vi "Create New Waypoint Dictionary ConfigFile.vi"() -> ()   [LabVIEW 2020, in "WyPtDict.lvlib"]
uses:
  WyPtDict.lvlib
  RoboWaypointDict Node--cluster.ctl
  BRS_Dev/Source Code/Robo Driver/Controls/MC and Robo Handshake.ctl
  StockerExpansionModuleID--enum.ctl
panel:
  out "Error":bool
  out "Nodes Written":i32=78
  out "error out":errorcluster={"status"=TRUE, "code"=10, "source"="Open/Create/Replace File in Easy Write XML File__JKI EasyXML.vi:3150001->Create New Waypoint Dictionary ConfigFile.vi<APPEND>\nC:\\Projects\\BRS-Dev\\BRS Information\\Waypoint Dictionary Configuration File.xml"}
  in  "error in (no error)":errorcluster
  in  "Waypoint Dictionary ConfigFile":path=path "C:/Projects/BRS-Dev/BRS Information/Waypoint Dictionary Configuration File - Template.xml"
  in  "WaypointDictionary":cluster{"WyPtDictNode":T1[]}={"WyPtDictNode"=[{"MC and Robo Handshake"=enum."None", "Idx"=0, "Cmd Number"="", "Waypoint List"="", "Description"="", "ExpMod ID"=enum."None"}, {"MC and Robo Handshake"=enum."Move and Pick Nikon Ret LP(1100)", "Idx"=1, "Cmd Number"="1100", "Waypoint List"="", "Description"="", "ExpMod ID"=enum."None"}, {"MC and Robo Handshake"=enum."Nikon Barcode1 Scanning Started(1101)", "Idx"=2, "Cmd Number"="1101", "Waypoint List"="", "Description"="", "ExpMod ID"=enum."None"}, {"MC and Robo Handshake"=enum."Nikon Barcode1 Scan Abort(1102)", "Idx"=3, "Cmd Number"="1102", "Waypoint List"="", "Description"="", "ExpMod ID"=enum."None"}, {"MC and Robo Handshake"=enum."Nikon Barcode1 Scan Success Proc to Barcode 2 Pos(1103)", "Idx"=4, "Cmd Number"="1103", "Waypoint List"="", "Description"="", "ExpMod ID"=enum."None"}, {"MC and Robo Handshake"=enum."Nikon Barcode 2 Scanning Started(1104)", "Idx"=5, "Cmd Number"="1104", "Waypoint List"="", "Description"="", "ExpMod ID"=enum."None"}, {"MC and Robo Handshake"=enum."Nikon Barcode 2 Scan Abort(1105) ", "Idx"=6, "Cmd Number"="1105", "Waypoint List"="", "Description"="", "ExpMod ID"=enum."None"}, {"MC and Robo Handshake"=enum."Nikon Barcode 2 Success(1106)", "Idx"=7, "Cmd Number"="1106", "Waypoint List"="", "Description"="", "ExpMod ID"=enum."None"}, {"MC and Robo Handshake"=enum."Move and Pick POZZ Ret LP(1300)", "Idx"=8, "Cmd Number"="1300", "Waypoint List"="", "Description"="", "ExpMod ID"=enum."None"}, {"MC and Robo Handshake"=enum."POZZ Barcode Scan Started(1301)", "Idx"=9, "Cmd Number"="1301", "Waypoint List"="", "Description"="", "ExpMod ID"=enum."None"}, {"MC and Robo Handshake"=enum."POZZ Barcode Not Found(1302)", "Idx"=10, "Cmd Number"="1302", "Waypoint List"="", "Description"="", "ExpMod ID"=enum."None"}, {"MC and Robo Handshake"=enum."POZZ Barcode Scan Succ(1303)", "Idx"=11, "Cmd Number"="1303", "Waypoint List"="", "Description"="", "ExpMod ID"=enum."None"}, {"MC and Robo Handshake"=enum."POZZ Mov to Side 2 Bar 2(1310)", "Idx"=12, "Cmd Number"="1310", "Waypoint List"="", "Description"="", "ExpMod ID"=enum."None"}, {"MC and Robo Handshake"=enum."POZZ Mov to Side 4 Bar 1(1311)", "Idx"=13, "Cmd Number"="1311", "Waypoint List"="", "Description"="", "ExpMod ID"=enum."None"}, {"MC and Robo Handshake"=enum."POZZ Mov to Side 4 Bar 2(1312)", "Idx"=14, "Cmd Number"="1312", "Waypoint List"="", "Description"="", "ExpMod ID"=enum."None"}, {"MC and Robo Handshake"=enum."POZZ Mov to Side 1 Bar 1(1313)", "Idx"=15, "Cmd Number"="1313", "Waypoint List"="", "Description"="", "ExpMod ID"=enum."None"}, {"MC and Robo Handshake"=enum."POZZ Mov to Side 1 Bar 2(1314)", "Idx"=16, "Cmd Number"="1314", "Waypoint List"="", "Description"="", "ExpMod ID"=enum."None"}, {"MC and Robo Handshake"=enum."POZZ Mov to Side 3 Bar 1(1315)", "Idx"=17, "Cmd Number"="1315", "Waypoint List"="", "Description"="", "ExpMod ID"=enum."None"}, {"MC and Robo Handshake"=enum."POZZ Mov to Side 3 Bar 2(1316)", "Idx"=18, "Cmd Number"="1316", "Waypoint List"="", "Description"="", "ExpMod ID"=enum."None"}, {"MC and Robo Handshake"=enum."POZZ Mov to Edge 3 Nik 2(1317)", "Idx"=19, "Cmd Number"="1317", "Waypoint List"="", "Description"="", "ExpMod ID"=enum."None"}, {"MC and Robo Handshake"=enum."POZZ Mov to Edge 4 ASML(1318)", "Idx"=20, "Cmd Number"="1318", "Waypoint List"="", "Description"="", "ExpMod ID"=enum."None"}, {"MC and Robo Handshake"=enum."POZZ Mov to Edge 4 Nik 1(1319)", "Idx"=21, "Cmd Number"="1319", "Waypoint List"="", "Description"="", "ExpMod ID"=enum."None"}, {"MC and Robo Handshake"=enum."POZZ Mov to Edge 4 Nik 2(1320)", "Idx"=22, "Cmd Number"="1320", "Waypoint List"="", "Description"="", "ExpMod ID"=enum."None"}, {"MC and Robo Handshake"=enum."Move to ASML LP and Pick Ret(2000)", "Idx"=23, "Cmd Number"="2000", "Waypoint List"="", "Description"="", "ExpMod ID"=enum."None"}, {"MC and Robo Handshake"=enum."ASML1 Barcode Scan Started(2001)", "Idx"=24, "Cmd Number"="2001", "Waypoint List"="", "Description"="", "ExpMod ID"=enum."None"}, {"MC and Robo Handshake"=enum."ASML1 Barcode Not Found(2002)", "Idx"=25, "Cmd Number"="2002", "Waypoint List"="", "Description"="", "ExpMod ID"=enum."None"}, {"MC and Robo Handshake"=enum."ASML1 Barcode Scan Succ(2003)", "Idx"=26, "Cmd Number"="2003", "Waypoint List"="", "Description"="", "ExpMod ID"=enum."None"}, {"MC and Robo Handshake"=enum."Start Load Seq for Nikon LP(3000)", "Idx"=27, "Cmd Number"="3000", "Waypoint List"="", "Description"="", "ExpMod ID"=enum."None"}, {"MC and Robo Handshake"=enum."Start Load Seq for POZZ LP(3200)", "Idx"=28, "Cmd Number"="3200", "Waypoint List"="", "Description"="", "ExpMod ID"=enum."None"}, {"MC and Robo Handshake"=enum."Start Load Seq for ASML LP(3400)", "Idx"=29, "Cmd Number"="3400", "Waypoint List"="", "Description"="", "ExpMod ID"=enum."None"}, {"MC and Robo Handshake"=enum."Start Align End Grip Place Func(4000)", "Idx"=30, "Cmd Number"="4000", "Waypoint List"="", "Description"="", "ExpMod ID"=enum."None"}, {"MC and Robo Handshake"=enum."Start Align End grip Pick Func(4001)", "Idx"=31, "Cmd Number"="4001", "Waypoint List"="", "Description"="", "ExpMod ID"=enum."None"}, {"MC and Robo Handshake"=enum."Start Align Center Grip Place Func(4002)", "Idx"=32, "Cmd Number"="4002", "Waypoint List"="", "Description"="", "ExpMod ID"=enum."None"}, {"MC and Robo Handshake"=enum."Start Align Center grip Pick Func(4003)", "Idx"=33, "Cmd Number"="4003", "Waypoint List"="", "Description"="", "ExpMod ID"=enum."None"}, {"MC and Robo Handshake"=enum."Start Move from home to Cleaner(5000)", "Idx"=34, "Cmd Number"="5000", "Waypoint List"="", "Description"="", "ExpMod ID"=enum."None"}, {"MC and Robo Handshake"=enum."Start Move to Final Cleaner Loc(5001)", "Idx"=35, "Cmd Number"="5001", "Waypoint List"="", "Description"="", "ExpMod ID"=enum."None"}, {"MC and Robo Handshake"=enum."Start Move from Cleaner loc to home(5002)", "Idx"=36, "Cmd Number"="5002", "Waypoint List"="", "Description"="", "ExpMod ID"=enum."None"}, {"MC and Robo Handshake"=enum."Start Move from home to PDS for Inspect(6000) ", "Idx"=37, "Cmd Number"="6000", "Waypoint List"="", "Description"="", "ExpMod ID"=enum."None"}, {"MC and Robo Handshake"=enum."PDS Inspect Finished(6001)", "Idx"=38, "Cmd Number"="6001", "Waypoint List"="", "Description"="", "ExpMod ID"=enum."None"}, {"MC and Robo Handshake"=enum."PDS EMO Recovery(6002)", "Idx"=39, "Cmd Number"="6002", "Waypoint List"="", "Description"="", "ExpMod ID"=enum."None"}, {"MC and Robo Handshake"=enum."Store in Stocker(7001)", "Idx"=40, "Cmd Number"="7001", "Waypoint List"="", "Description"="", "ExpMod ID"=enum."None"}, {"MC and Robo Handshake"=enum."Store in Expansion Stocker(7402)", "Idx"=41, "Cmd Number"="7401", "Waypoint List"="", "Description"="", "ExpMod ID"=enum."None"}, {"MC and Robo Handshake"=enum."Retrive from Center Stocker(8001)", "Idx"=42, "Cmd Number"="8001", "Waypoint List"="", "Description"="", "ExpMod ID"=enum."None"}, {"MC and Robo Handshake"=enum."Retrive Mov to Nikon BC1 Scan Pos(8002)", "Idx"=43, "Cmd Number"="8002", "Waypoint List"="", "Description"="", "ExpMod ID"=enum."None"}, {"MC and Robo Handshake"=enum."Retrive Nikon BC1not found(8003)", "Idx"=44, "Cmd Number"="8003", "Waypoint List"="", "Description"="", "ExpMod ID"=enum."None"}, {"MC and Robo Handshake"=enum."Retrive Nikon BC1 Scan Succ(8004)", "Idx"=45, "Cmd Number"="8004", "Waypoint List"="", "Description"="", "ExpMod ID"=enum."None"}, {"MC and Robo Handshake"=enum."Retrive Nikon BC2 not found(8005)", "Idx"=46, "Cmd Number"="8005", "Waypoint List"="", "Description"="", "ExpMod ID"=enum."None"}, {"MC and Robo Handshake"=enum."Retrive Nikon BC2 scan Succ(8006)", "Idx"=47, "Cmd Number"="8006", "Waypoint List"="", "Description"="", "ExpMod ID"=enum."None"}, {"MC and Robo Handshake"=enum."Retrive Mov to Edge 1 ASML(8202) ", "Idx"=48, "Cmd Number"="8202", "Waypoint List"="", "Description"="", "ExpMod ID"=enum."None"}, {"MC and Robo Handshake"=enum."Retrive Mov to Edge 1 Nikon 1(8203)", "Idx"=49, "Cmd Number"="8203", "Waypoint List"="", "Description"="", "ExpMod ID"=enum."None"}, {"MC and Robo Handshake"=enum."Retrive Mov to Edge 1 Nikon 2(8204)", "Idx"=50, "Cmd Number"="8204", "Waypoint List"="", "Description"="", "ExpMod ID"=enum."None"}, {"MC and Robo Handshake"=enum."Retrive Mov to Edge 2 ASML(8205)", "Idx"=51, "Cmd Number"="8205", "Waypoint List"="", "Description"="", "ExpMod ID"=enum."None"}, {"MC and Robo Handshake"=enum."Retrive Mov to Edge 2 Nikon 1(8206)", "Idx"=52, "Cmd Number"="8206", "Waypoint List"="", "Description"="", "ExpMod ID"=enum."None"}, {"MC and Robo Handshake"=enum."Retrive Mov to Edge 2 Nikon 2(8207)", "Idx"=53, "Cmd Number"="8207", "Waypoint List"="", "Description"="", "ExpMod ID"=enum."None"}, {"MC and Robo Handshake"=enum."Retrive Mov to Edge 3 ASML (8208)", "Idx"=54, "Cmd Number"="8208", "Waypoint List"="", "Description"="", "ExpMod ID"=enum."None"}, {"MC and Robo Handshake"=enum."Retrive Mov to Edge 3 Nikon 1(8209)", "Idx"=55, "Cmd Number"="8209", "Waypoint List"="", "Description"="", "ExpMod ID"=enum."None"}, {"MC and Robo Handshake"=enum."Retrive Mov to Edge 3 Nikon 2(8210)", "Idx"=56, "Cmd Number"="8210", "Waypoint List"="", "Description"="", "ExpMod ID"=enum."None"}, {"MC and Robo Handshake"=enum."Retrive Mov to Edge 4 ASML (8211)", "Idx"=57, "Cmd Number"="8211", "Waypoint List"="", "Description"="", "ExpMod ID"=enum."None"}, {"MC and Robo Handshake"=enum."Retrive Mov to Edge 4 Nikon 1 (8212)", "Idx"=58, "Cmd Number"="8212", "Waypoint List"="", "Description"="", "ExpMod ID"=enum."None"}, {"MC and Robo Handshake"=enum."Retrive Mov to Edge 4 Nikon 2 (8213)", "Idx"=59, "Cmd Number"="8213", "Waypoint List"="", "Description"="", "ExpMod ID"=enum."None"}, {"MC and Robo Handshake"=enum."Retrive BC Scan Abort (8214)", "Idx"=60, "Cmd Number"="8214", "Waypoint List"="", "Description"="", "ExpMod ID"=enum."None"}, {"MC and Robo Handshake"=enum."Retrive BC Scan Successful (8215)", "Idx"=61, "Cmd Number"="8215", "Waypoint List"="", "Description"="", "ExpMod ID"=enum."None"}, {"MC and Robo Handshake"=enum."Retrive Mov to ASML BC scan Pos (8402) ", "Idx"=62, "Cmd Number"="8402", "Waypoint List"="", "Description"="", "ExpMod ID"=enum."None"}, {"MC and Robo Handshake"=enum."Retrive ASML BC not found(8403)", "Idx"=63, "Cmd Number"="8403", "Waypoint List"="", "Description"="", "ExpMod ID"=enum."None"}, {"MC and Robo Handshake"=enum."Retrive ASML BC Scan Succ(8404)", "Idx"=64, "Cmd Number"="8404", "Waypoint List"="", "Description"="", "ExpMod ID"=enum."None"}, {"MC and Robo Handshake"=enum."Expansion Retrive Seq (8602)", "Idx"=65, "Cmd Number"="8601", "Waypoint List"="", "Description"="", "ExpMod ID"=enum."None"}, {"MC and Robo Handshake"=enum."Cen Stocker move from home to Transit Nest(9000)", "Idx"=66, "Cmd Number"="9000", "Waypoint List"="", "Description"="", "ExpMod ID"=enum."None"}, {"MC and Robo Handshake"=enum."Cen Stocker move from Transit Nest to home(9200)", "Idx"=67, "Cmd Number"="9200", "Waypoint List"="", "Description"="", "ExpMod ID"=enum."None"}, {"MC and Robo Handshake"=enum."Exp Stocker move from home to Transit Nest(9400)", "Idx"=68, "Cmd Number"="9400", "Waypoint List"="", "Description"="", "ExpMod ID"=enum."None"}, {"MC and Robo Handshake"=enum."Exp Stocker move from Transit Nest to home(9600)", "Idx"=69, "Cmd Number"="9600", "Waypoint List"="", "Description"="", "ExpMod ID"=enum."None"}, {"MC and Robo Handshake"=enum."Move to R1 Home (1000)", "Idx"=70, "Cmd Number"="1000", "Waypoint List"="", "Description"="", "ExpMod ID"=enum."None"}, {"MC and Robo Handshake"=enum."Move to R2 Home (1111)", "Idx"=71, "Cmd Number"="1000", "Waypoint List"="", "Description"="", "ExpMod ID"=enum."None"}, {"MC and Robo Handshake"=enum."Store Left Stocker (7401)", "Idx"=72, "Cmd Number"="7401", "Waypoint List"="", "Description"="", "ExpMod ID"=enum."None"}, {"MC and Robo Handshake"=enum."Retrieve Left Stocker (8601)", "Idx"=73, "Cmd Number"="8601", "Waypoint List"="", "Description"="", "ExpMod ID"=enum."None"}, {"MC and Robo Handshake"=enum."EMO Recovery Center (1002)", "Idx"=74, "Cmd Number"="1002", "Waypoint List"="", "Description"="", "ExpMod ID"=enum."None"}, {"MC and Robo Handshake"=enum."EMO Recovery Right (1003)", "Idx"=75, "Cmd Number"="1002", "Waypoint List"="", "Description"="", "ExpMod ID"=enum."None"}, {"MC and Robo Handshake"=enum."Center Robo Status (8888)", "Idx"=76, "Cmd Number"="8888", "Waypoint List"="", "Description"="", "ExpMod ID"=enum."None"}, {"MC and Robo Handshake"=enum."Right Robo Status (8889)", "Idx"=77, "Cmd Number"="8888", "Waypoint List"="", "Description"="", "ExpMod ID"=enum."None"}]}
  # "XML Configuration File"
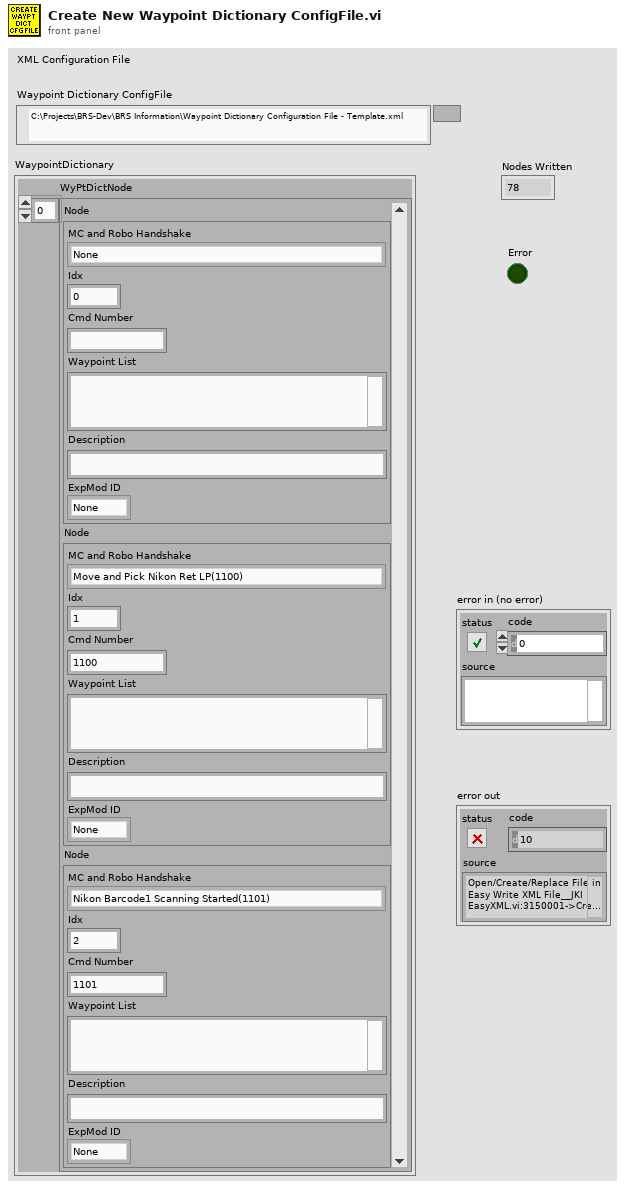
[diagram p1: front panel]
types:
  T1 = typedef "WyPtDict.lvlib/RoboWaypointDict Node--cluster.ctl" = cluster{"MC and Robo Handshake":T2, "Idx":i32, "Cmd Number":string, "Waypoint List":string, "Description":string, "ExpMod ID":T3}
  T2 = typedef "MC and Robo Handshake.ctl" = enum16{"None", "Move and Pick Nikon Ret LP(1100)", "Nikon Barcode1 Scanning Started(1101)", "Nikon Barcode1 Scan Abort(1102)", "Nikon Barcode1 Scan Success Proc to Barcode 2 Pos(1103)", "Nikon Barcode 2 Scanning Started(1104)", "Nikon Barcode 2 Scan Abort(1105) ", "Nikon Barcode 2 Success(1106)", "Move and Pick POZZ Ret LP(1300)", "POZZ Barcode Scan Started(1301)", "POZZ Barcode Not Found(1302)", "POZZ Barcode Scan Succ(1303)", "POZZ Mov to Side 2 Bar 2(1310)", "POZZ Mov to Side 4 Bar 1(1311)", "POZZ Mov to Side 4 Bar 2(1312)", "POZZ Mov to Side 1 Bar 1(1313)", "POZZ Mov to Side 1 Bar 2(1314)", "POZZ Mov to Side 3 Bar 1(1315)", "POZZ Mov to Side 3 Bar 2(1316)", "POZZ Mov to Edge 3 Nik 2(1317)", "POZZ Mov to Edge 4 ASML(1318)", "POZZ Mov to Edge 4 Nik 1(1319)", "POZZ Mov to Edge 4 Nik 2(1320)", "Move to ASML LP and Pick Ret(2000)", "ASML1 Barcode Scan Started(2001)", "ASML1 Barcode Not Found(2002)", "ASML1 Barcode Scan Succ(2003)", "Start Load Seq for Nikon LP(3000)", "Start Load Seq for POZZ LP(3200)", "Start Load Seq for ASML LP(3400)", "Start Align End Grip Place Func(4000)", "Start Align End grip Pick Func(4001)", "Start Align Center Grip Place Func(4002)", "Start Align Center grip Pick Func(4003)", "Start Move from home to Cleaner(5000)", "Start Move to Final Cleaner Loc(5001)", "Start Move from Cleaner loc to home(5002)", "Start Move from home to PDS for Inspect(6000) ", "PDS Inspect Finished(6001)", "PDS EMO Recovery(6002)", "Store in Stocker(7001)", "Store in Expansion Stocker(7402)", "Retrive from Center Stocker(8001)", "Retrive Mov to Nikon BC1 Scan Pos(8002)", "Retrive Nikon BC1not found(8003)", "Retrive Nikon BC1 Scan Succ(8004)", "Retrive Nikon BC2 not found(8005)", "Retrive Nikon BC2 scan Succ(8006)", "Retrive Mov to Edge 1 ASML(8202) ", "Retrive Mov to Edge 1 Nikon 1(8203)", "Retrive Mov to Edge 1 Nikon 2(8204)", "Retrive Mov to Edge 2 ASML(8205)", "Retrive Mov to Edge 2 Nikon 1(8206)", "Retrive Mov to Edge 2 Nikon 2(8207)", "Retrive Mov to Edge 3 ASML (8208)", "Retrive Mov to Edge 3 Nikon 1(8209)", "Retrive Mov to Edge 3 Nikon 2(8210)", "Retrive Mov to Edge 4 ASML (8211)", "Retrive Mov to Edge 4 Nikon 1 (8212)", "Retrive Mov to Edge 4 Nikon 2 (8213)", "Retrive BC Scan Abort (8214)", "Retrive BC Scan Successful (8215)", "Retrive Mov to ASML BC scan Pos (8402) ", "Retrive ASML BC not found(8403)", "Retrive ASML BC Scan Succ(8404)", "Expansion Retrive Seq (8602)", "Cen Stocker move from home to Transit Nest(9000)", "Cen Stocker move from Transit Nest to home(9200)", "Exp Stocker move from home to Transit Nest(9400)", "Exp Stocker move from Transit Nest to home(9600)", "Move to R1 Home (1000)", "Move to R2 Home (1111)", "Store Left Stocker (7401)", "Retrieve Left Stocker (8601)", "EMO Recovery Center (1002)", "EMO Recovery Right (1003)", "Center Robo Status (8888)", "Right Robo Status (8889)"}
  T3 = typedef "WyPtDict.lvlib/StockerExpansionModuleID--enum.ctl" = enum16{"None", "Main", "Exp1", "Exp2", "Exp3", "Exp4", "Exp5"}
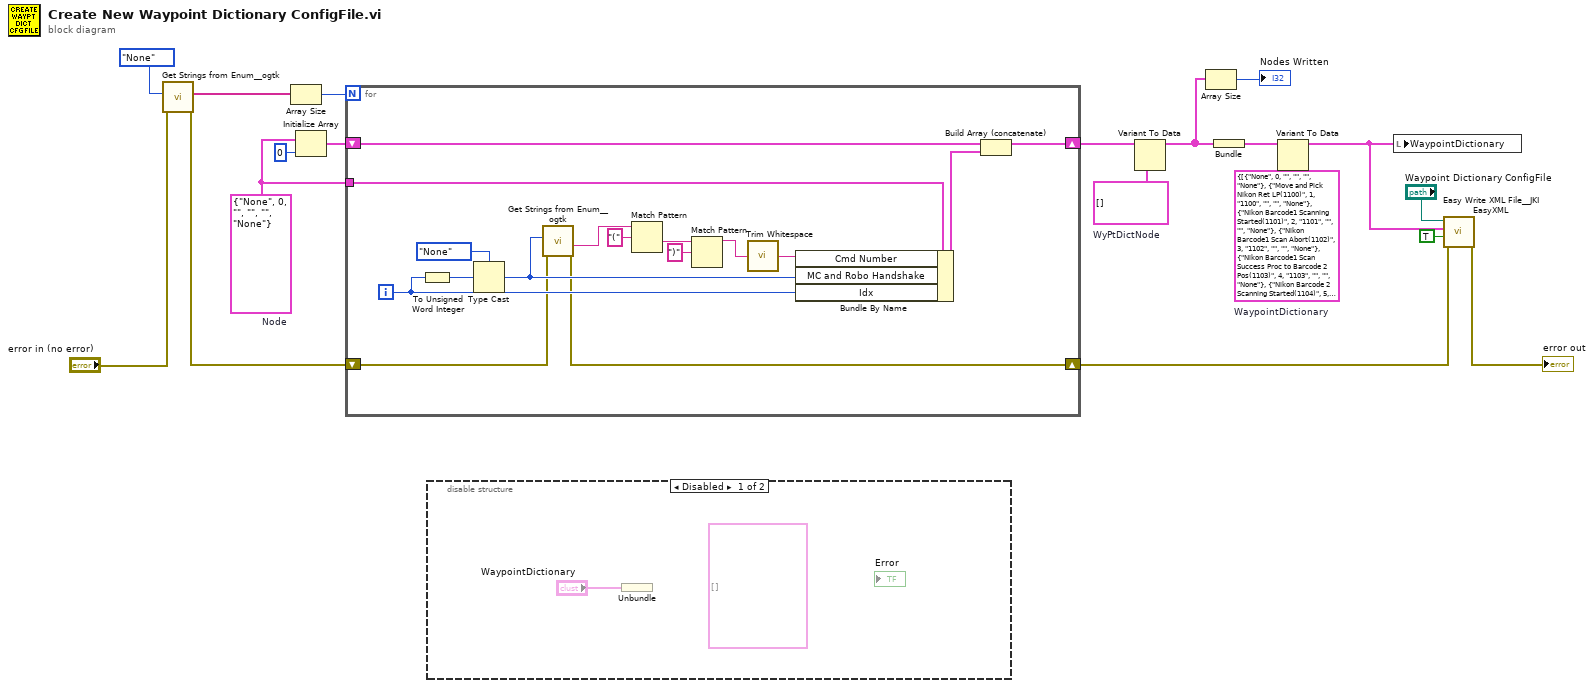
[diagram p0: block diagram]
diagram:
  w2 = cluster{"WyPtDictNode":T1[]} {"WyPtDictNode"=[{"MC and Robo Handshake"=enum."None", "Idx"=0, "Cmd Number"="", "Waypoint List"="", "Description"="", "ExpMod ID"=enum."None"}, {"MC and Robo Handshake"=enum."Move and Pick Nikon Ret LP(1100)", "Idx"=1, "Cmd Number"="1100", "Waypoint List"="", "Description"="", "ExpMod ID"=enum."None"}, {"MC and Robo Handshake"=enum."Nikon Barcode1 Scanning Started(1101)", "Idx"=2, "Cmd Number"="1101", "Waypoint List"="", "Description"="", "ExpMod ID"=enum."None"}, {"MC and Robo Handshake"=enum."Nikon Barcode1 Scan Abort(1102)", "Idx"=3, "Cmd Number"="1102", "Waypoint List"="", "Description"="", "ExpMod ID"=enum."None"}, {"MC and Robo Handshake"=enum."Nikon Barcode1 Scan Success Proc to Barcode 2 Pos(1103)", "Idx"=4, "Cmd Number"="1103", "Waypoint List"="", "Description"="", "ExpMod ID"=enum."None"}, {"MC and Robo Handshake"=enum."Nikon Barcode 2 Scanning Started(1104)", "Idx"=5, "Cmd Number"="1104", "Waypoint List"="", "Description"="", "ExpMod ID"=enum."None"}, {"MC and Robo Handshake"=enum."Nikon Barcode 2 Scan Abort(1105) ", "Idx"=6, "Cmd Number"="1105", "Waypoint List"="", "Description"="", "ExpMod ID"=enum."None"}, {"MC and Robo Handshake"=enum."Nikon Barcode 2 Success(1106)", "Idx"=7, "Cmd Number"="1106", "Waypoint List"="", "Description"="", "ExpMod ID"=enum."None"}, {"MC and Robo Handshake"=enum."Move and Pick POZZ Ret LP(1300)", "Idx"=8, "Cmd Number"="1300", "Waypoint List"="", "Description"="", "ExpMod ID"=enum."None"}, {"MC and Robo Handshake"=enum."POZZ Barcode Scan Started(1301)", "Idx"=9, "Cmd Number"="1301", "Waypoint List"="", "Description"="", "ExpMod ID"=enum."None"}, {"MC and Robo Handshake"=enum."POZZ Barcode Not Found(1302)", "Idx"=10, "Cmd Number"="1302", "Waypoint List"="", "Description"="", "ExpMod ID"=enum."None"}, {"MC and Robo Handshake"=enum."POZZ Barcode Scan Succ(1303)", "Idx"=11, "Cmd Number"="1303", "Waypoint List"="", "Description"="", "ExpMod ID"=enum."None"}, {"MC and Robo Handshake"=enum."POZZ Mov to Side 2 Bar 2(1310)", "Idx"=12, "Cmd Number"="1310", "Waypoint List"="", "Description"="", "ExpMod ID"=enum."None"}, {"MC and Robo Handshake"=enum."POZZ Mov to Side 4 Bar 1(1311)", "Idx"=13, "Cmd Number"="1311", "Waypoint List"="", "Description"="", "ExpMod ID"=enum."None"}, {"MC and Robo Handshake"=enum."POZZ Mov to Side 4 Bar 2(1312)", "Idx"=14, "Cmd Number"="1312", "Waypoint List"="", "Description"="", "ExpMod ID"=enum."None"}, {"MC and Robo Handshake"=enum."POZZ Mov to Side 1 Bar 1(1313)", "Idx"=15, "Cmd Number"="1313", "Waypoint List"="", "Description"="", "ExpMod ID"=enum."None"}, {"MC and Robo Handshake"=enum."POZZ Mov to Side 1 Bar 2(1314)", "Idx"=16, "Cmd Number"="1314", "Waypoint List"="", "Description"="", "ExpMod ID"=enum."None"}, {"MC and Robo Handshake"=enum."POZZ Mov to Side 3 Bar 1(1315)", "Idx"=17, "Cmd Number"="1315", "Waypoint List"="", "Description"="", "ExpMod ID"=enum."None"}, {"MC and Robo Handshake"=enum."POZZ Mov to Side 3 Bar 2(1316)", "Idx"=18, "Cmd Number"="1316", "Waypoint List"="", "Description"="", "ExpMod ID"=enum."None"}, {"MC and Robo Handshake"=enum."POZZ Mov to Edge 3 Nik 2(1317)", "Idx"=19, "Cmd Number"="1317", "Waypoint List"="", "Description"="", "ExpMod ID"=enum."None"}, {"MC and Robo Handshake"=enum."POZZ Mov to Edge 4 ASML(1318)", "Idx"=20, "Cmd Number"="1318", "Waypoint List"="", "Description"="", "ExpMod ID"=enum."None"}, {"MC and Robo Handshake"=enum."POZZ Mov to Edge 4 Nik 1(1319)", "Idx"=21, "Cmd Number"="1319", "Waypoint List"="", "Description"="", "ExpMod ID"=enum."None"}, {"MC and Robo Handshake"=enum."POZZ Mov to Edge 4 Nik 2(1320)", "Idx"=22, "Cmd Number"="1320", "Waypoint List"="", "Description"="", "ExpMod ID"=enum."None"}, {"MC and Robo Handshake"=enum."Move to ASML LP and Pick Ret(2000)", "Idx"=23, "Cmd Number"="2000", "Waypoint List"="", "Description"="", "ExpMod ID"=enum."None"}, {"MC and Robo Handshake"=enum."ASML1 Barcode Scan Started(2001)", "Idx"=24, "Cmd Number"="2001", "Waypoint List"="", "Description"="", "ExpMod ID"=enum."None"}, {"MC and Robo Handshake"=enum."ASML1 Barcode Not Found(2002)", "Idx"=25, "Cmd Number"="2002", "Waypoint List"="", "Description"="", "ExpMod ID"=enum."None"}, {"MC and Robo Handshake"=enum."ASML1 Barcode Scan Succ(2003)", "Idx"=26, "Cmd Number"="2003", "Waypoint List"="", "Description"="", "ExpMod ID"=enum."None"}, {"MC and Robo Handshake"=enum."Start Load Seq for Nikon LP(3000)", "Idx"=27, "Cmd Number"="3000", "Waypoint List"="", "Description"="", "ExpMod ID"=enum."None"}, {"MC and Robo Handshake"=enum."Start Load Seq for POZZ LP(3200)", "Idx"=28, "Cmd Number"="3200", "Waypoint List"="", "Description"="", "ExpMod ID"=enum."None"}, {"MC and Robo Handshake"=enum."Start Load Seq for ASML LP(3400)", "Idx"=29, "Cmd Number"="3400", "Waypoint List"="", "Description"="", "ExpMod ID"=enum."None"}, {"MC and Robo Handshake"=enum."Start Align End Grip Place Func(4000)", "Idx"=30, "Cmd Number"="4000", "Waypoint List"="", "Description"="", "ExpMod ID"=enum."None"}, {"MC and Robo Handshake"=enum."Start Align End grip Pick Func(4001)", "Idx"=31, "Cmd Number"="4001", "Waypoint List"="", "Description"="", "ExpMod ID"=enum."None"}, {"MC and Robo Handshake"=enum."Start Align Center Grip Place Func(4002)", "Idx"=32, "Cmd Number"="4002", "Waypoint List"="", "Description"="", "ExpMod ID"=enum."None"}, {"MC and Robo Handshake"=enum."Start Align Center grip Pick Func(4003)", "Idx"=33, "Cmd Number"="4003", "Waypoint List"="", "Description"="", "ExpMod ID"=enum."None"}, {"MC and Robo Handshake"=enum."Start Move from home to Cleaner(5000)", "Idx"=34, "Cmd Number"="5000", "Waypoint List"="", "Description"="", "ExpMod ID"=enum."None"}, {"MC and Robo Handshake"=enum."Start Move to Final Cleaner Loc(5001)", "Idx"=35, "Cmd Number"="5001", "Waypoint List"="", "Description"="", "ExpMod ID"=enum."None"}, {"MC and Robo Handshake"=enum."Start Move from Cleaner loc to home(5002)", "Idx"=36, "Cmd Number"="5002", "Waypoint List"="", "Description"="", "ExpMod ID"=enum."None"}, {"MC and Robo Handshake"=enum."Start Move from home to PDS for Inspect(6000) ", "Idx"=37, "Cmd Number"="6000", "Waypoint List"="", "Description"="", "ExpMod ID"=enum."None"}, {"MC and Robo Handshake"=enum."PDS Inspect Finished(6001)", "Idx"=38, "Cmd Number"="6001", "Waypoint List"="", "Description"="", "ExpMod ID"=enum."None"}, {"MC and Robo Handshake"=enum."PDS EMO Recovery(6002)", "Idx"=39, "Cmd Number"="6002", "Waypoint List"="", "Description"="", "ExpMod ID"=enum."None"}, {"MC and Robo Handshake"=enum."Store in Stocker(7001)", "Idx"=40, "Cmd Number"="7001", "Waypoint List"="", "Description"="", "ExpMod ID"=enum."None"}, {"MC and Robo Handshake"=enum."Store in Expansion Stocker(7402)", "Idx"=41, "Cmd Number"="7401", "Waypoint List"="", "Description"="", "ExpMod ID"=enum."None"}, {"MC and Robo Handshake"=enum."Retrive from Center Stocker(8001)", "Idx"=42, "Cmd Number"="8001", "Waypoint List"="", "Description"="", "ExpMod ID"=enum."None"}, {"MC and Robo Handshake"=enum."Retrive Mov to Nikon BC1 Scan Pos(8002)", "Idx"=43, "Cmd Number"="8002", "Waypoint List"="", "Description"="", "ExpMod ID"=enum."None"}, {"MC and Robo Handshake"=enum."Retrive Nikon BC1not found(8003)", "Idx"=44, "Cmd Number"="8003", "Waypoint List"="", "Description"="", "ExpMod ID"=enum."None"}, {"MC and Robo Handshake"=enum."Retrive Nikon BC1 Scan Succ(8004)", "Idx"=45, "Cmd Number"="8004", "Waypoint List"="", "Description"="", "ExpMod ID"=enum."None"}, {"MC and Robo Handshake"=enum."Retrive Nikon BC2 not found(8005)", "Idx"=46, "Cmd Number"="8005", "Waypoint List"="", "Description"="", "ExpMod ID"=enum."None"}, {"MC and Robo Handshake"=enum."Retrive Nikon BC2 scan Succ(8006)", "Idx"=47, "Cmd Number"="8006", "Waypoint List"="", "Description"="", "ExpMod ID"=enum."None"}, {"MC and Robo Handshake"=enum."Retrive Mov to Edge 1 ASML(8202) ", "Idx"=48, "Cmd Number"="8202", "Waypoint List"="", "Description"="", "ExpMod ID"=enum."None"}, {"MC and Robo Handshake"=enum."Retrive Mov to Edge 1 Nikon 1(8203)", "Idx"=49, "Cmd Number"="8203", "Waypoint List"="", "Description"="", "ExpMod ID"=enum."None"}, {"MC and Robo Handshake"=enum."Retrive Mov to Edge 1 Nikon 2(8204)", "Idx"=50, "Cmd Number"="8204", "Waypoint List"="", "Description"="", "ExpMod ID"=enum."None"}, {"MC and Robo Handshake"=enum."Retrive Mov to Edge 2 ASML(8205)", "Idx"=51, "Cmd Number"="8205", "Waypoint List"="", "Description"="", "ExpMod ID"=enum."None"}, {"MC and Robo Handshake"=enum."Retrive Mov to Edge 2 Nikon 1(8206)", "Idx"=52, "Cmd Number"="8206", "Waypoint List"="", "Description"="", "ExpMod ID"=enum."None"}, {"MC and Robo Handshake"=enum."Retrive Mov to Edge 2 Nikon 2(8207)", "Idx"=53, "Cmd Number"="8207", "Waypoint List"="", "Description"="", "ExpMod ID"=enum."None"}, {"MC and Robo Handshake"=enum."Retrive Mov to Edge 3 ASML (8208)", "Idx"=54, "Cmd Number"="8208", "Waypoint List"="", "Description"="", "ExpMod ID"=enum."None"}, {"MC and Robo Handshake"=enum."Retrive Mov to Edge 3 Nikon 1(8209)", "Idx"=55, "Cmd Number"="8209", "Waypoint List"="", "Description"="", "ExpMod ID"=enum."None"}, {"MC and Robo Handshake"=enum."Retrive Mov to Edge 3 Nikon 2(8210)", "Idx"=56, "Cmd Number"="8210", "Waypoint List"="", "Description"="", "ExpMod ID"=enum."None"}, {"MC and Robo Handshake"=enum."Retrive Mov to Edge 4 ASML (8211)", "Idx"=57, "Cmd Number"="8211", "Waypoint List"="", "Description"="", "ExpMod ID"=enum."None"}, {"MC and Robo Handshake"=enum."Retrive Mov to Edge 4 Nikon 1 (8212)", "Idx"=58, "Cmd Number"="8212", "Waypoint List"="", "Description"="", "ExpMod ID"=enum."None"}, {"MC and Robo Handshake"=enum."Retrive Mov to Edge 4 Nikon 2 (8213)", "Idx"=59, "Cmd Number"="8213", "Waypoint List"="", "Description"="", "ExpMod ID"=enum."None"}, {"MC and Robo Handshake"=enum."Retrive BC Scan Abort (8214)", "Idx"=60, "Cmd Number"="8214", "Waypoint List"="", "Description"="", "ExpMod ID"=enum."None"}, {"MC and Robo Handshake"=enum."Retrive BC Scan Successful (8215)", "Idx"=61, "Cmd Number"="8215", "Waypoint List"="", "Description"="", "ExpMod ID"=enum."None"}, {"MC and Robo Handshake"=enum."Retrive Mov to ASML BC scan Pos (8402) ", "Idx"=62, "Cmd Number"="8402", "Waypoint List"="", "Description"="", "ExpMod ID"=enum."None"}, {"MC and Robo Handshake"=enum."Retrive ASML BC not found(8403)", "Idx"=63, "Cmd Number"="8403", "Waypoint List"="", "Description"="", "ExpMod ID"=enum."None"}, {"MC and Robo Handshake"=enum."Retrive ASML BC Scan Succ(8404)", "Idx"=64, "Cmd Number"="8404", "Waypoint List"="", "Description"="", "ExpMod ID"=enum."None"}, {"MC and Robo Handshake"=enum."Expansion Retrive Seq (8602)", "Idx"=65, "Cmd Number"="8601", "Waypoint List"="", "Description"="", "ExpMod ID"=enum."None"}, {"MC and Robo Handshake"=enum."Cen Stocker move from home to Transit Nest(9000)", "Idx"=66, "Cmd Number"="9000", "Waypoint List"="", "Description"="", "ExpMod ID"=enum."None"}, {"MC and Robo Handshake"=enum."Cen Stocker move from Transit Nest to home(9200)", "Idx"=67, "Cmd Number"="9200", "Waypoint List"="", "Description"="", "ExpMod ID"=enum."None"}, {"MC and Robo Handshake"=enum."Exp Stocker move from home to Transit Nest(9400)", "Idx"=68, "Cmd Number"="9400", "Waypoint List"="", "Description"="", "ExpMod ID"=enum."None"}, {"MC and Robo Handshake"=enum."Exp Stocker move from Transit Nest to home(9600)", "Idx"=69, "Cmd Number"="9600", "Waypoint List"="", "Description"="", "ExpMod ID"=enum."None"}, {"MC and Robo Handshake"=enum."Move to R1 Home (1000)", "Idx"=70, "Cmd Number"="1000", "Waypoint List"="", "Description"="", "ExpMod ID"=enum."None"}, {"MC and Robo Handshake"=enum."Move to R2 Home (1111)", "Idx"=71, "Cmd Number"="1000", "Waypoint List"="", "Description"="", "ExpMod ID"=enum."None"}, {"MC and Robo Handshake"=enum."Store Left Stocker (7401)", "Idx"=72, "Cmd Number"="7401", "Waypoint List"="", "Description"="", "ExpMod ID"=enum."None"}, {"MC and Robo Handshake"=enum."Retrieve Left Stocker (8601)", "Idx"=73, "Cmd Number"="8601", "Waypoint List"="", "Description"="", "ExpMod ID"=enum."None"}, {"MC and Robo Handshake"=enum."EMO Recovery Center (1002)", "Idx"=74, "Cmd Number"="1002", "Waypoint List"="", "Description"="", "ExpMod ID"=enum."None"}, {"MC and Robo Handshake"=enum."EMO Recovery Right (1003)", "Idx"=75, "Cmd Number"="1002", "Waypoint List"="", "Description"="", "ExpMod ID"=enum."None"}, {"MC and Robo Handshake"=enum."Center Robo Status (8888)", "Idx"=76, "Cmd Number"="8888", "Waypoint List"="", "Description"="", "ExpMod ID"=enum."None"}, {"MC and Robo Handshake"=enum."Right Robo Status (8889)", "Idx"=77, "Cmd Number"="8888", "Waypoint List"="", "Description"="", "ExpMod ID"=enum."None"}]}  # WaypointDictionary
  w3 = T1[] []  # WyPtDictNode
  w15 = T1 {"MC and Robo Handshake"=enum."None", "Idx"=0, "Cmd Number"="", "Waypoint List"="", "Description"="", "ExpMod ID"=enum."None"}  # Node
  n1 = call <userlib>:"Get Strings from Enum__ogtk.vi"("error in (no error)"="error in (no error)", "Enum"=MC_and_Robo_Handshake."None" ("MC and Robo Handshake")) -> ("error out"=w11:errorcluster, "Enum Strings"=w17:string[])  [unwired: 6 in, 2 out]
  n2 = Array Size(array=w17) -> (size(s)=w14:i32)
  n3 = Initialize Array(w15, 0 ("dimension size")) -> (w19:T1[])
  n4 = for {
    N: w14 -> [_]
    shift-right: [w31] -> w4
    shift-left: w19 -> [w33]
    tunnel: w15 -> [w34]
    shift-right: [w22] -> w8
    shift-left: w11 -> [w23]
    i -> [w30]
    n5 = To Unsigned Word Integer(number=w30) -> (unsigned 16bit integer=w29:u16)
    n6 = Type Cast(type=MC_and_Robo_Handshake."None" ("MC and Robo Handshake"), x=w29) -> (*(type *) &x=w28:T2)
    n7 = call <userlib>:"Get Strings from Enum__ogtk.vi"("error in (no error)"=w23, "Enum"=w28) -> ("error out"=w22:errorcluster, "String Value"=w21:string)  [unwired: 6 in, 2 out]
    n8 = Match Pattern(string=w21, regular expression="(") -> (after substring=w26:string)  [unwired: 1 in, 3 out]
    n9 = Match Pattern(string=w26, regular expression=")") -> (before substring=w24:string)  [unwired: 1 in, 3 out]
    n10 = call <vilib>:"Trim Whitespace.vi"("string"=w24) -> ("trimmed string"=w20:string)  [unwired: 1 in]
    n11 = Bundle By Name(cluster=w34, "Cmd Number"=w20, "MC and Robo Handshake"=w28, "Idx"=w30) -> (w32:T1)
    n12 = Build Array (concatenate)(w33, w32) -> (w31:T1[])
  }
  n13 = disable-structure shown="Disabled" {
    frame Disabled {
      (unwired) T1[] [] ("WyPtDictNode Array")
      n14 = Unbundle("WaypointDictionary") -> ()  [unwired: 1 out]
    }
    frame Enabled {
    }
  }
  n15 = Variant To Data(type=w3, Variant=w4) -> (data=w5:T1[])  [unwired: 1 in, 1 out]
  n16 = Array Size(array=w5) -> (size(s)=→"Nodes Written":i32)
  n17 = Bundle("WyPtDictNode"=w5) -> (w9:cluster{"WyPtDictNode":T1[]})  [unwired: 1 in]
  n18 = Variant To Data(type=w2, Variant=w9) -> (data=w1:cluster{"WyPtDictNode":T1[]})  [unwired: 1 in, 1 out]
  n19 = local write "WaypointDictionary"(w1) -> ()
  n20 = call <vilib>:"Easy Write XML File__JKI EasyXML.vi"("error in (no error)"=w8, "Overwrite File? (false)"=TRUE, "LabVIEW Data"=w1, "XML File Path"="Waypoint Dictionary ConfigFile") -> ("error out"=→"error out":errorcluster)  [unwired: 6 in, 1 out]
